vi "IBM4_Diff_Read(IN).vi"(7 "Number":i32=10, 8 "error in":errorcluster, 9 "Neg-Chan":i32=1, 10 "Pos-Chan":i32, 11 "COM resource in":refnum<visa-resource-name>="COM9") -> (0 "error out":errorcluster, 2 "array":i32[](array[numeric]), 3 "COM resource out":refnum<visa-resource-name>)   [LabVIEW 2021, in "IBM4.lvlib"]
doc: "This VI interfaces with the IBM4 to perform a differential read operation.\n\nThe input channels must be between 0 and 4, and the number of readings should be greater than zero. At some point the number of reading will be too high and will cause a timeout error. This should only happen for numbers larger than 10000. The output will be an array of integer values.\n\nAlternate read operations exist covering binary or floating point, single reading, multiple readings, and an average of multiple readings (floating point only)."
uses:
  <instrlib>/IBM4/IBM4.lvlib
  <vilib>/regexp/Match Regular Expression.xnode
panel:
  out "error out 2":errorcluster
  out "read buffer":string
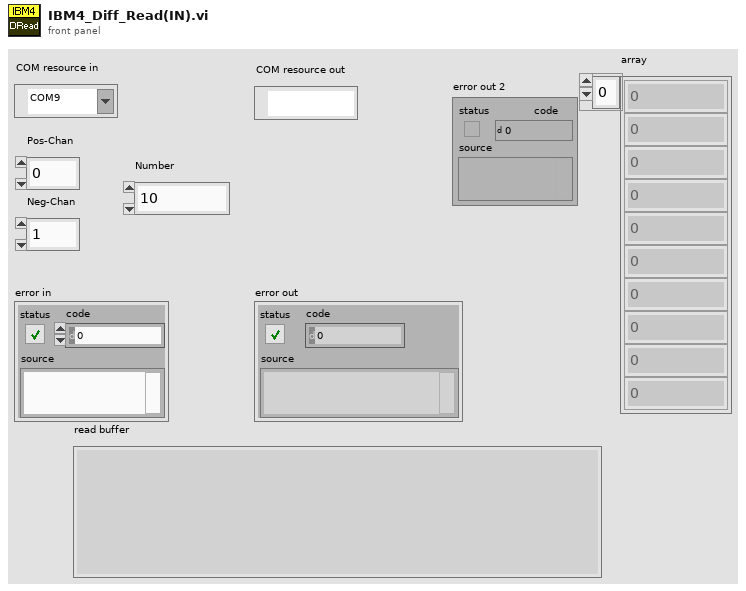
[diagram p1: front panel]
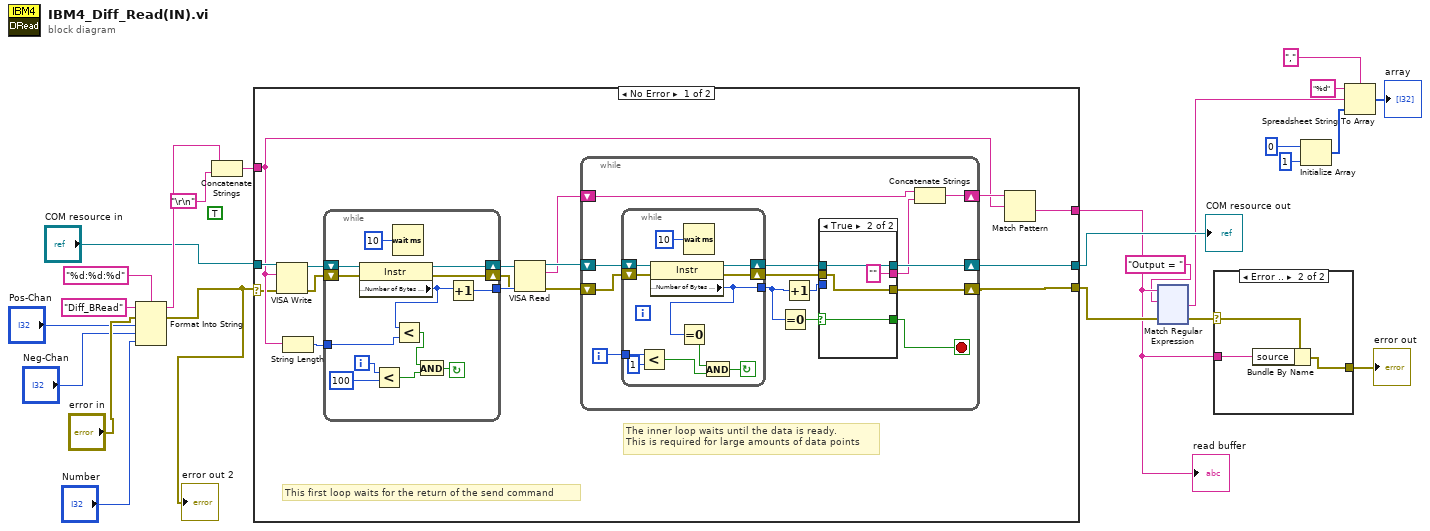
[diagram p0: block diagram]
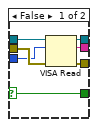
[diagram p3: hidden frame]
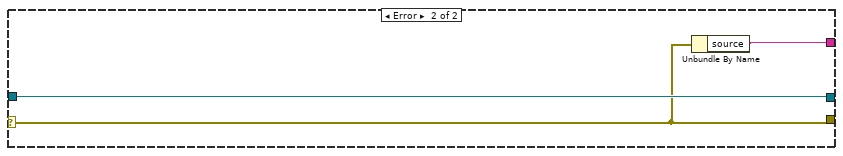
[diagram p4: hidden frame]
diagram:
  (unwired) TRUE ("Enable Termination\nChar (T)")
  n1 = Format Into String(format string="%d:%d:%d", initial string="Diff_BRead", error in="error in", "Pos-Chan", "Neg-Chan", "Number") -> (resulting string=w18:string, error out=w1:errorcluster)
  "error out 2" <- w1
  n2 = Concatenate Strings(w18, "\r\n") -> (w17:string)
  n3 = case shown="No Error" w1 {
    selector: w1 -> [w27 w90]
    tunnel: "COM resource in" -> [w40 w92]
    tunnel: [w26 w90] -> w7
    tunnel: [w38 w91] -> w5
    tunnel: w17 -> [w37 _]
    tunnel: [w25 w92] -> w20
    frame No Error {
      # "The inner loop waits until the data is ready.\nThis is required for large amounts of data points"
      # "This first loop waits for the return of the send command"
      n4 = VISA Write(VISA resource name=w40, write buffer=w37, error in (no error)=w27) -> (VISA resource name out=w36:refnum<visa-resource-name>, error out=w35:errorcluster)  [unwired: 1 out]
      n5 = String Length(string=w37) -> (length=w28:i32)
      n6 = while {
        tunnel: [w42] -> w33
        shift-right: [w52] -> w34
        shift-left: w36 -> [w53]
        shift-right: [w50] -> w32
        shift-left: w35 -> [w51]
        tunnel: w28 -> [w48]
        i -> [w43]
        stop <- w46 continue-if-true
        n7 = property class="Instr"(reference=w53, error in=w51) -> (reference out=w52:refnum<visa-resource-name>, error out=w50:errorcluster, "Serial Settings:Number of Bytes at Serial Port"=w41:u32)
        n8 = Less?(x=w43, y=100) -> (x < y?=w45:bool)
        n9 = Wait (ms)(milliseconds to wait=u32 10) -> ()  [unwired: 1 out]
        n10 = Less?(x=w41, y=w48) -> (x < y?=w44:bool)
        n11 = And(x=w44, y=w45) -> (x .and. y?=w46:bool)
        n12 = Increment(x=w41) -> (x+1=w42:u32)
      }
      n13 = VISA Read(VISA resource name=w34, byte count=w33, error in (no error)=w32) -> (VISA resource name out=w31:refnum<visa-resource-name>, read buffer=w29:string, error out=w30:errorcluster)  [unwired: 1 out]
      n14 = while {
        shift-right: [w67] -> w25
        shift-left: w31 -> [w65]
        shift-right: [w66] -> w26
        shift-left: w30 -> [w63]
        shift-right: [w61] -> w39
        shift-left: w29 -> [w59]
        i -> [w58]
        stop <- w54 stop-if-true
        n15 = while {
          tunnel: [w84] -> w57
          shift-right: [w88] -> w64
          shift-left: w65 -> [w89]
          shift-right: [w86] -> w62
          shift-left: w63 -> [w87]
          tunnel: w58 -> [w83]
          stop <- w81 continue-if-true
          n16 = Less?(x=w83, y=1) -> (x < y?=w80:bool)
          n17 = property class="Instr"(reference=w89, error in=w87) -> (reference out=w88:refnum<visa-resource-name>, error out=w86:errorcluster, "Serial Settings:Number of Bytes at Serial Port"=w84:u32)
          n18 = Equal To 0?(x=w84) -> (x = 0?=w79:bool)
          n19 = Wait (ms)(milliseconds to wait=u32 10) -> ()  [unwired: 1 out]
          n20 = And(x=w79, y=w80) -> (x .and. y?=w81:bool)
        }
        n21 = Equal To 0?(x=w57) -> (x = 0?=w55:bool)
        n22 = Increment(x=w57) -> (x+1=w56:u32)
        n23 = case shown="True" w55 {
          selector: w55 -> [w68 w77]
          tunnel: [w74 w78] -> w67
          tunnel: [w73 w76] -> w66
          tunnel: w64 -> [w72 w78]
          tunnel: w62 -> [w71 w76]
          tunnel: [w70 "" ("read buffer")] -> w60
          tunnel: w56 -> [w69 _]
          tunnel: [w68 w77] -> w54
          frame False {
            n24 = VISA Read(VISA resource name=w72, byte count=w69, error in (no error)=w71) -> (VISA resource name out=w74:refnum<visa-resource-name>, read buffer=w70:string, error out=w73:errorcluster)  [unwired: 1 out]
          }
          frame True {
          }
        }
        n25 = Concatenate Strings(w59, w60) -> (w61:string)
      }
      n26 = Match Pattern(string=w39, regular expression=w37) -> (after substring=w38:string)  [unwired: 1 in, 3 out]
    }
    frame Error {
      n27 = Unbundle By Name(w90) -> ("source"=w91:string)
    }
  }
  "COM resource out" <- w20
  "read buffer" <- w5
  n28 = xnode "Match Regular Expression"("input string"=w5, "regular expression"="Output = " ("format string"), "error in"=w7) -> ("after match"=w3:string, "error out"=w6:errorcluster)  [unwired: 3 in, 3 out]
  n29 = case shown="Error .." w6 {
    selector: w6 -> [w93 w96]
    tunnel: [w93 w94] -> w16
    tunnel: w5 -> [_ w95]
    frame No Error {
    }
    frame Error {
      n30 = Bundle By Name(cluster=w96, "source"=w95) -> (w94:errorcluster)
    }
  }
  "error out" <- w16
  n31 = Initialize Array(0, 1 ("dimension size")) -> (w12:i32[])
  n32 = Spreadsheet String To Array(delimiter (Tab)=",", format string="%d", spreadsheet string=w3, array type (2D Dbl)=w12) -> (array=→"array":i32[])
